vi "Open.vi"(8 "error in (no error)":errorcluster, 11 "LibreVNA in":refnum<class "LibreVNA.lvclass">) -> (0 "error out":errorcluster, 3 "LibreVNA out":refnum<class "LibreVNA.lvclass">)   [LabVIEW 2023, in "LibreVNA.lvclass"]
uses:
  LibreVNA.lvclass
  LibreVNA.lvclass/LibreVNA.ctl
panel:
  out "IsOpen":bool
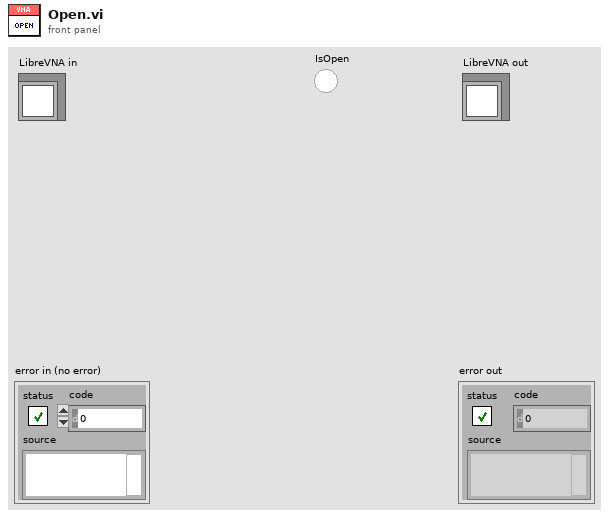
[diagram p1: front panel]
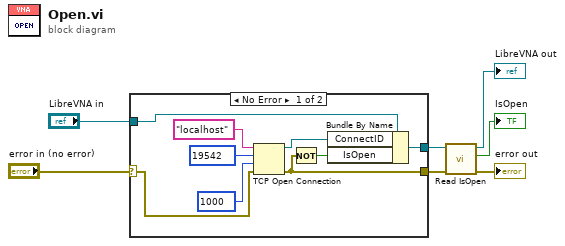
[diagram p0: block diagram]
diagram:
  n1 = case shown="No Error" "error in (no error)" {
    selector: "error in (no error)" -> [w11 w18]
    tunnel: [w9 w18] -> w2
    tunnel: [w13 w17] -> w5
    tunnel: "LibreVNA in" -> [w16 w17]
    frame No Error {
      n2 = TCP Open Connection(address="localhost", remote port or service name=u16 19542, timeout ms (60000)=1000, error in (no error)=w11) -> (connection ID=w12:refnum<k5>, error out=w9:errorcluster)  [unwired: 1 in]
      n3 = Not(x=w9) -> (.not. x?=w8:bool)
      n4 = Bundle By Name(cluster=w16, "ConnectID"=w12, "IsOpen"=w8) -> (w13:refnum<class "LibreVNA.lvclass">)
    }
    frame Error {
    }
  }
  n5 = call-dynamic "Read IsOpen.vi"("error in (no error)"=w2, "LibreVNA in"=w5) -> ("error out"=→"error out":errorcluster, "IsOpen"=→"IsOpen":bool, "LibreVNA out"=→"LibreVNA out":refnum<class "LibreVNA.lvclass">)  [unwired: 7 in]
